vi "Send Voltage Limit.vi"(8 "error in":errorcluster, 11 "89XX in":refnum<class "89XX.lvclass">) -> (0 "error out":errorcluster, 3 "89XX out":refnum<class "89XX.lvclass">)   [LabVIEW 2019, in "89XX.lvlib" / "89XX.lvclass"]
uses:
  Library/89XX.lvclass
  C:/Users/Public/Documents/Development/builds/Instruments/PowerSupply.lvlibp/Library/PowerSupply.lvclass
  Library/89XX.lvclass/89XX.ctl
  Accessors/Read Local Resource.vi
  <instrlib>/Keysight N8900 Series/Keysight N8900 Series.lvlib
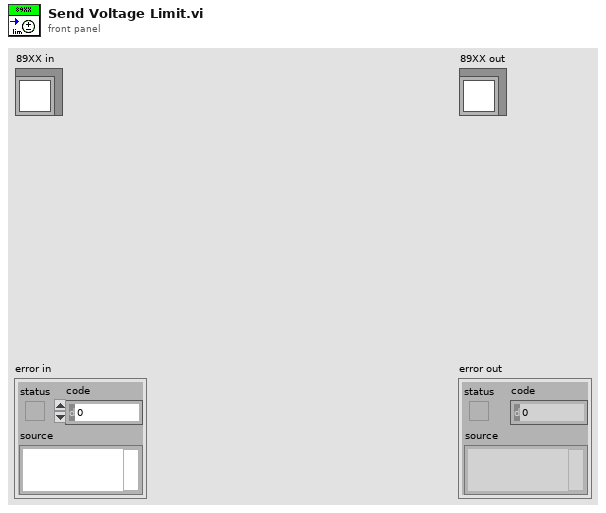
[diagram p1: front panel]
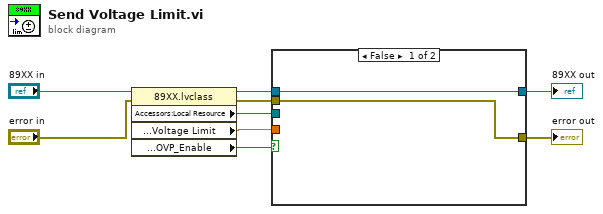
[diagram p0: block diagram]
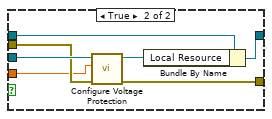
[diagram p2: hidden frame]
diagram:
  n1 = property class="89XX.lvclass"(reference="89XX in", error in="error in") -> (reference out=w7:refnum<class "89XX.lvclass">, error out=w4:errorcluster, "Accessors:Local Resource"=w5:refnum<visa-resource-name>, "Accessors:Setting:Protection:Voltage Limit"=w2:dbl, "Accessors:Setting:Protection:OVP_Enable"=w1:bool)
  n2 = case shown="False" w1 {
    tunnel: w7 -> [w11 w18]
    tunnel: [w11 w17] -> w6
    tunnel: w5 -> [_ w15]
    tunnel: w4 -> [w10 w14]
    tunnel: [w10 w13] -> w3
    tunnel: w2 -> [_ w12]
    frame False {
    }
    frame True {
      n3 = call <instrlib>:"Configure Voltage Protection.vi"("error in (no error)"=w14, "Protection Level (96 volts)"=w12, "VISA resource name"=w15) -> ("error out"=w13:errorcluster, "VISA resource name out"=w16:refnum<visa-resource-name>)  [unwired: 7 in]
      n4 = Bundle By Name(cluster=w18, "Local Resource"=w16) -> (w17:refnum<class "89XX.lvclass">)
    }
  }
  "error out" <- w3
  "89XX out" <- w6
